vi "First Array Element [String].vi"(2 "Array":string[](array[string])) -> (7 "First Element":string)   [LabVIEW 2019]
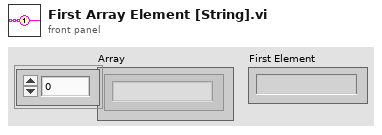
[diagram p1: front panel]
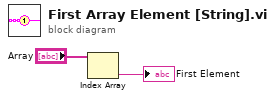
[diagram p0: block diagram]
diagram:
  n1 = Index Array(array="Array") -> (element=→"First Element":string)  [unwired: 1 in]
